vi "AlliGator Gate Image File Name Format Dialog.vi"(8 "error in (no error)":errorcluster, 9 "Single Image":bool, 10 "Saved TIFF Image":T1=enum."Sum of All Gates" caption="Displayed Image", 11 "Image File Name in":string) -> (0 "error out":errorcluster, 1 "Start Index out":u32 caption="Start Index", 2 "File Number Format out":string caption="File Number Format", 3 "Gate Image File Name out":string caption="Image File Name", 4 "Compress Image out":bool caption="Compress Image", 5 "Cancelled?":bool, 6 "Save Metadata File out":bool caption="Save Metadata File")   [LabVIEW 2021, in "AlliGator Files.lvlib"]
doc: "Dialog to specify naming convention for gate image files (or other image files)."
uses:
  AlliGator Files.lvlib
  AlliGator Saved TIFF Image Type.ctl
panel:
  in  "Compress Image":bool
  in  "Start Index":u32 format="%0.0f"
  in  "Save Metadata File":bool
  in  "File Number Format":string
  in  "File Name":string caption="Gate Image File Name"
  out "String":string="Enter TIFF File Name and numbering format:"
  in  "Cancel":bool
  in  "OK":bool caption="OK2"
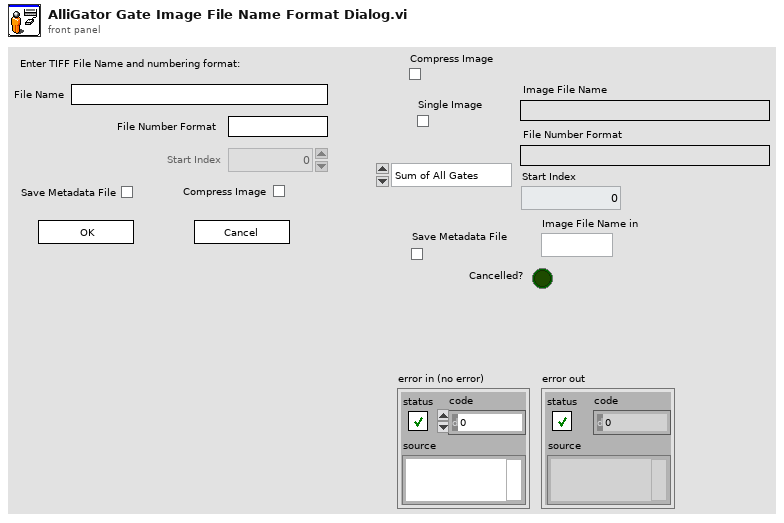
[diagram p1: front panel]
types:
  T1 = typedef "AlliGator Files.lvlib/AlliGator Saved TIFF Image Type.ctl" = enum16{"Single Gate", "Sum of All Gates", "Phasor"}
  T2 = enum8{"Enabled", "Disabled", "Disabled and Grayed Out"}
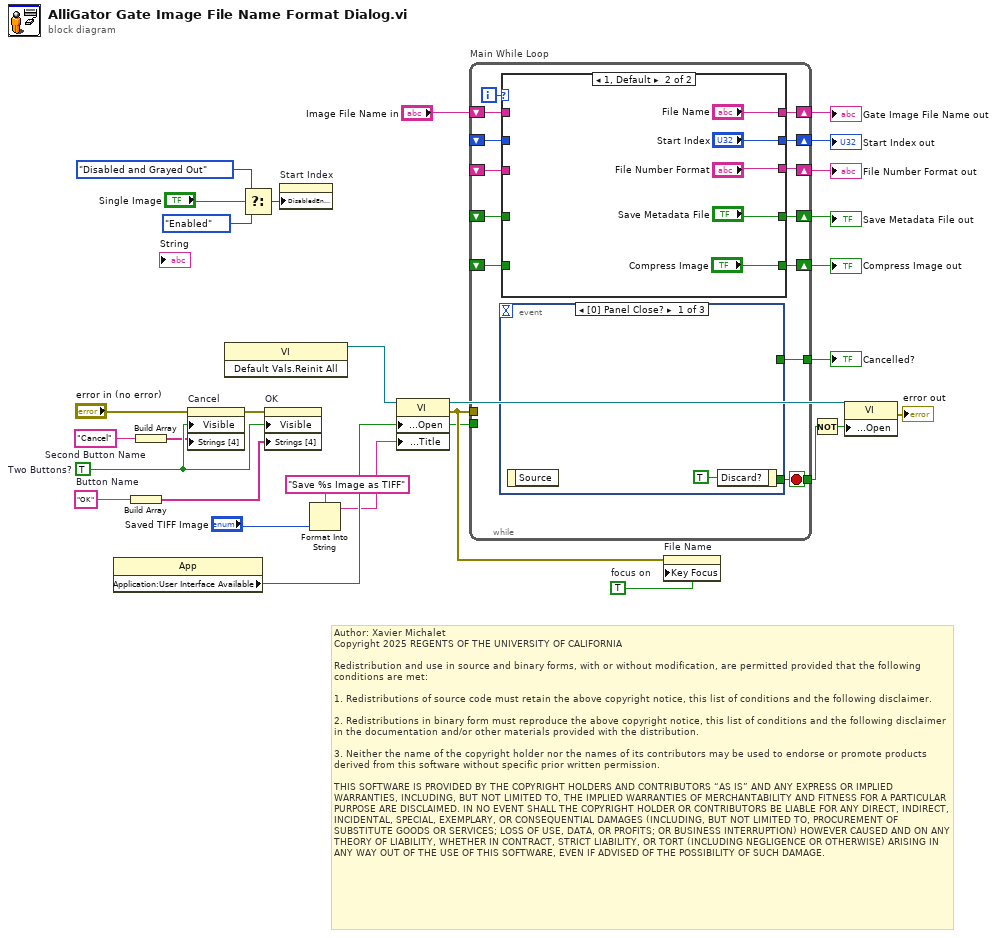
[diagram p0: block diagram]
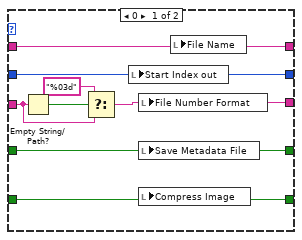
[diagram p2: hidden frame]
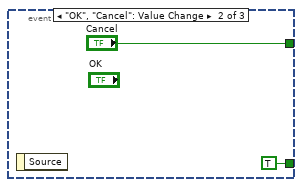
[diagram p3: hidden frame]
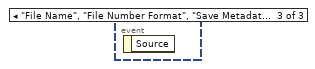
[diagram p4: hidden frame]
diagram:
  w17 = TRUE  # focus on
  w25 = "Cancel"  # Second Button Name
  w23 = "OK"  # Button Name
  w29 = TRUE  # Two Buttons?
  # "Author: Xavier Michalet\nCopyright 2025 REGENTS OF THE UNIVERSITY OF CALIFORNIA\n\nRedistribution and use in source and binary forms, with or without modification, are permitted provided that the following conditions are met:\n\n1. Redistributions of source code must retain the above copyright notice, this list of conditions and the following disclaimer.\n\n2. Redistributions in binary form must reproduce the above copyright notice, this list of conditions and the following disclaimer in the documentation and/or other materials provided with the distribution.\n\n3. Neither the name of the copyright holder nor the names of its contributors may be used to endorse or promote products derived from this software without specific prior written permission.\n\nTHIS SOFTWARE IS PROVIDED BY THE COPYRIGHT HOLDERS AND CONTRIBUTORS “AS IS” AND ANY EXPRESS OR IMPLIED WARRANTIES, INCLUDING, BUT NOT LIMITED TO, THE IMPLIED WARRANTIES OF MERCHANTABILITY AND FITNESS FOR A PARTICULAR PURPOSE ARE DISCLAIMED. IN NO EVENT SHALL THE COPYRIGHT HOLDER OR CONTRIBUTORS BE LIABLE FOR ANY DIRECT, INDIRECT, INCIDENTAL, SPECIAL, EXEMPLARY, OR CONSEQUENTIAL DAMAGES (INCLUDING, BUT NOT LIMITED TO, PROCUREMENT OF SUBSTITUTE GOODS OR SERVICES; LOSS OF USE, DATA, OR PROFITS; OR BUSINESS INTERRUPTION) HOWEVER CAUSED AND ON ANY THEORY OF LIABILITY, WHETHER IN CONTRACT, STRICT LIABILITY, OR TORT (INCLUDING NEGLIGENCE OR OTHERWISE) ARISING IN ANY WAY OUT OF THE USE OF THIS SOFTWARE, EVEN IF ADVISED OF THE POSSIBILITY OF SUCH DAMAGE."
  n1 = property class="App"() -> ("Application:User Interface Available"=w19:bool)  [unwired: 2 in, 2 out]
  n2 = Build Array(w23) -> (w24:string[])
  n3 = Build Array(w25) -> (w26:string[])
  n4 = property on="Cancel" class="Bool"(error in="error in (no error)", "Visible"=w29, "Strings [4]"=w26) -> (error out=w28:errorcluster)  [unwired: 1 in, 1 out]
  n5 = invoke class="VI" method="Default Vals.Reinit All"() -> (reference out=w18:refnum<vi>)  [unwired: 3 in, 2 out]
  n6 = Select(t=T2."Disabled and Grayed Out" ("Disabled"), s="Single Image", f=T2."Enabled" ("Disabled")) -> (s? t:f=w4:T2)
  n7 = property on="OK" class="Bool"(error in=w28, "Visible"=w29, "Strings [4]"=w24) -> ()  [unwired: 1 in, 2 out]
  n8 = property on="Start Index" class="DigNum (strict)"("DisabledEnum"=w4) -> ()  [unwired: 2 in, 2 out]
  n9 = Format Into String(format string="Save %s Image as TIFF", "Saved TIFF Image") -> (resulting string=w1:string)  [unwired: 2 in, 1 out]
  n10 = property class="VI"(reference=w18, "Front Panel Window:Open"=w19, "Front Panel.Title"=w1) -> (reference out=w10:refnum<vi>, error out=w22:errorcluster)  [unwired: 1 in]
  n11 = while "Main While Loop" {
    tunnel: w19 -> [_]
    tunnel: w22 -> [_]
    shift-right: [w38] -> w12
    shift-left: _ -> [w39]
    shift-right: [w36] -> w13
    shift-left: _ -> [w37]
    tunnel: [w42] -> w16
    shift-right: [w35] -> w14
    shift-left: "Image File Name in" -> [w40]
    tunnel: [w34] -> w11
    shift-right: [w33] -> w9
    shift-left: _ -> [w32]
    shift-right: [w31] -> w8
    shift-left: _ -> [w30]
    i -> [w41]
    stop <- w34 stop-if-true
    n12 = event shown="[0] Panel Close?" {
      selector: _ -> [_ _ _]
      dyn-events: _ -> [_ _ _]
      timeout: _ -> [_ _ _]
      tunnel: [w56 TRUE ("Discard?") _] -> w34
      tunnel: [_ "Cancel" _] -> w42
      event Panel Close? {
        w56 = TRUE ("Discard?")
        n13 = event-data() -> ()  [unwired: 1 in, 1 out]
        n14 = event-data("Discard?"=w56) -> ()  [unwired: 1 in, 1 out]
      }
      event "OK", "Cancel": Value Change {
        n15 = event-data() -> ()  [unwired: 1 in, 1 out]
      }
      event "File Name", "File Number Format", "Save Metadata File", "Start Index", "Compress Image": Value Change {
        n16 = event-data() -> ()  [unwired: 1 in, 1 out]
      }
    }
    n17 = case shown="1, Default" w41 {
      tunnel: w40 -> [w49 _]
      tunnel: w39 -> [w50 _]
      tunnel: [w50 "Save Metadata File"] -> w38
      tunnel: w37 -> [w43 _]
      tunnel: [w44 "File Number Format"] -> w36
      tunnel: [w49 "File Name"] -> w35
      tunnel: [w48 "Start Index"] -> w33
      tunnel: w32 -> [w48 _]
      tunnel: [w47 "Compress Image"] -> w31
      tunnel: w30 -> [w47 _]
      frame 0 {
        n18 = Empty String/Path?(string/path=w43) -> (empty?=w46:bool)
        n19 = Select(t="%03d" ("File Number Format"), s=w46, f=w43) -> (s? t:f=w44:string)
        n20 = local write "Start Index out"(w48) -> ()
        n21 = local write "File Number Format"(w44) -> ()
        n22 = local write "Save Metadata File"(w50) -> ()
        n23 = local write "Compress Image"(w47) -> ()
        n24 = local write "File Name"(w49) -> ()
      }
      frame 1, Default {
      }
    }
  }
  "Cancelled?" <- w16
  "Gate Image File Name out" <- w14
  "File Number Format out" <- w13
  "Save Metadata File out" <- w12
  "Start Index out" <- w9
  "Compress Image out" <- w8
  n25 = property on="File Name" class="Str"(error in=w22, "Key Focus"=w17) -> ()  [unwired: 1 in, 2 out]
  n26 = Not(x=w11) -> (.not. x?=w27:bool)
  n27 = property class="VI"(reference=w10, "Front Panel Window:Open"=w27) -> (error out=→"error out":errorcluster)  [unwired: 1 in, 1 out]
